vi "grayScreen.vi"(8 "error in (no error)":errorcluster, 11 "Stimulus in":refnum<class "Stimulus.lvclass">) -> (0 "error out":errorcluster, 3 "Stimulus out":refnum<class "Stimulus.lvclass">)   [LabVIEW 2014, in "Stimulus.lvclass"]
uses:
  Stimulus.lvclass
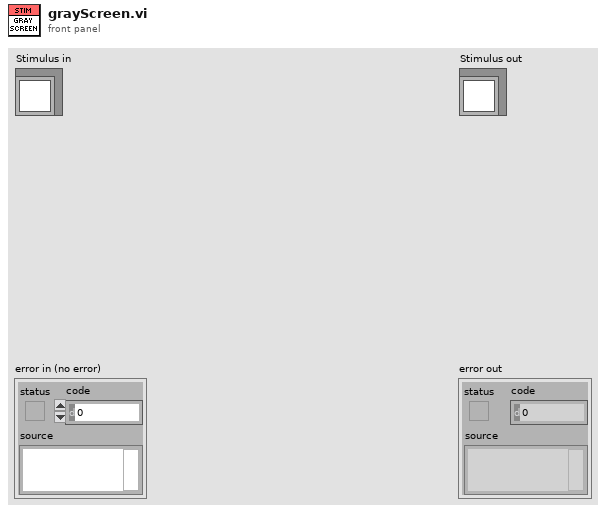
[diagram p1: front panel]
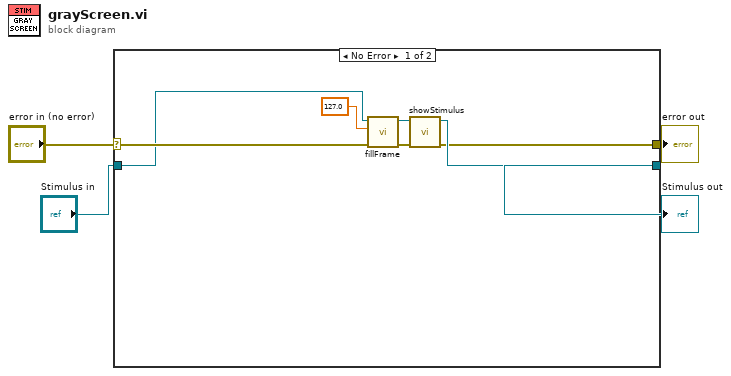
[diagram p0: block diagram]
diagram:
  n1 = case shown="No Error" "error in (no error)" {
    selector: "error in (no error)" -> [w9 w13]
    tunnel: [w10 w13] -> w3
    tunnel: [w11 w12] -> w1
    tunnel: "Stimulus in" -> [w8 w12]
    frame No Error {
      n2 = call-dynamic "fillFrame.vi"("error in (no error)"=w9, "Pixel Value (U8, U16, I16, Float)"=sgl 127.0, "Stimulus in"=w8) -> ("error out"=w5:errorcluster, "Stimulus out"=w6:refnum<class "Stimulus.lvclass">)  [unwired: 7 in]
      n3 = call-dynamic "showStimulus.vi"("error in (no error)"=w5, "Stimulus in"=w6) -> ("error out"=w10:errorcluster, "Stimulus out"=w11:refnum<class "Stimulus.lvclass">)  [unwired: 8 in]
    }
    frame Error {
    }
  }
  "error out" <- w3
  "Stimulus out" <- w1
